vi "AAL Resample (Const to Variable, multi-channel).vi"(7 "reset? (True)":bool=TRUE, 8 "error in (no error)":errorcluster, 9 "config":T1={"timing jitter"=enum."Interpolation", "anti-aliasing?"=TRUE, "filter prototype"={"coefficients"=[], "factor"=1}} {"filter prototype"."coefficients" format="%.2f"}, 10 "time":dbl[](array[numeric]) format="%.2f", 11 "X":dbl[][](array[numeric])) -> (0 "error out":errorcluster, 1 "offset":i32, 2 "time stamps":dbl[](array[numeric]) format="%.2f", 3 "Y":dbl[][](array[numeric]) format="%.2f")   [LabVIEW 2010, in "NI_AALPro.lvlib"]
doc: "Perform an arbitrary resampling on the input signal."
uses:
  NI_AALPro.lvlib
  lvanlys.dll
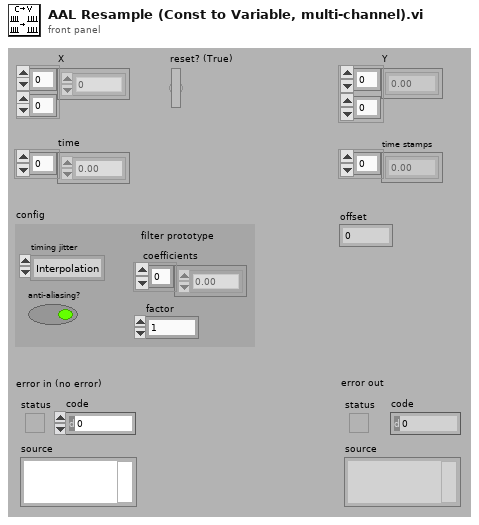
[diagram p1: front panel]
types:
  T1 = cluster{"timing jitter":enum32{"Interpolation", "Rounding"}, "anti-aliasing?":bool, "filter prototype":cluster{"coefficients":dbl[], "factor":i32}}
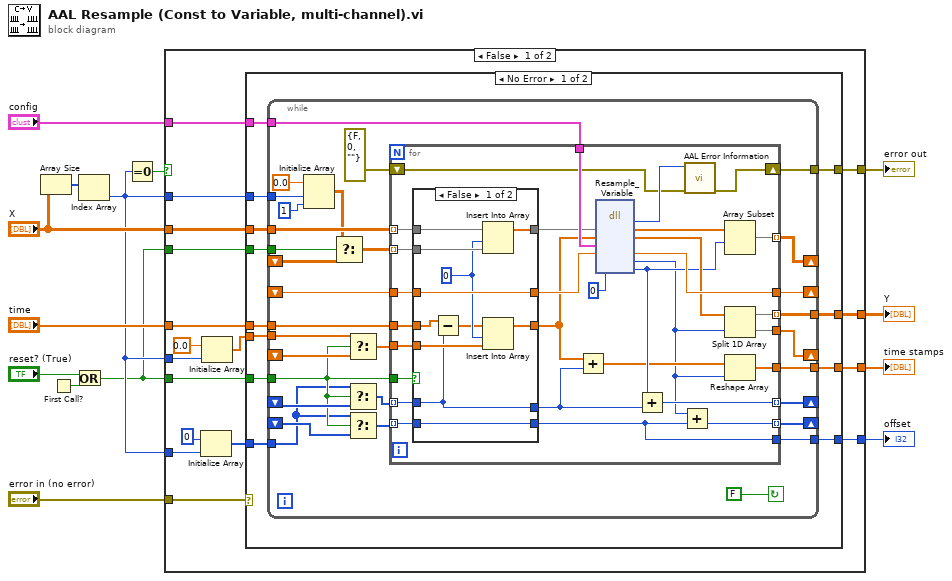
[diagram p0: block diagram]
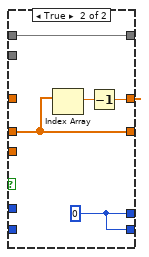
[diagram p2: hidden frame]
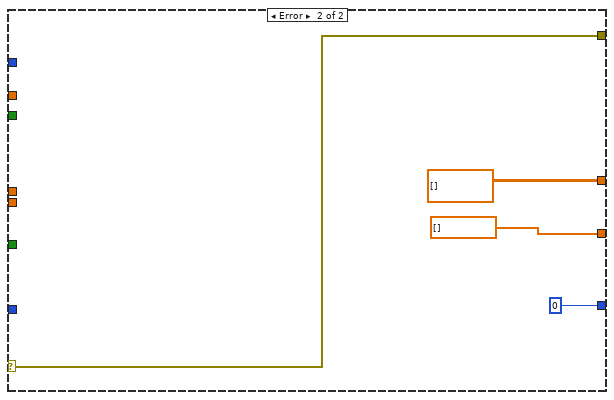
[diagram p3: hidden frame]
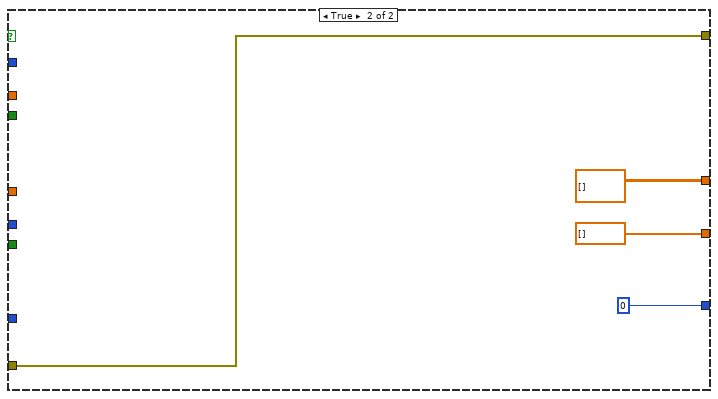
[diagram p4: hidden frame]
diagram:
  n1 = Array Size(array="X") -> (size(s)=w6:i32[])
  n2 = First Call?() -> (First Call?: T/F=w5:bool)
  n3 = Or(x="reset? (True)", y=w5) -> (x .or. y?=w1:bool)
  n4 = Index Array(array=w6) -> (element=w2:i32)  [unwired: 1 in]
  n5 = Equal To 0?(x=w2) -> (x = 0?=w3:bool)
  n6 = case shown="False" w3 {
    tunnel: "config" -> [w31 _]
    tunnel: "time" -> [w30 _]
    tunnel: [w29 dbl[] []] -> w12
    tunnel: [w28 dbl[][] []] -> w11
    tunnel: [w27 0 ("element")] -> w10
    tunnel: [w26 w126] -> w9
    tunnel: "error in (no error)" -> [w25 w126]
    tunnel: "X" -> [w24 _]
    tunnel: w1 -> [w21 _]
    tunnel: w2 -> [w19 _]
    tunnel: w2 -> [w17 _]
    tunnel: w2 -> [w16 _]
    tunnel: w1 -> [w15 _]
    frame False {
      n7 = Initialize Array(0 ("element"), w16) -> (w18:i32[])
      n8 = Initialize Array(0.0 ("element"), w17) -> (w20:dbl[])
      n9 = case shown="No Error" w25 {
        selector: w25 -> [_ w124]
        tunnel: w31 -> [w43 _]
        tunnel: w30 -> [w38 _]
        tunnel: [w42 dbl[] []] -> w29
        tunnel: [w41 dbl[][] []] -> w28
        tunnel: [w40 0] -> w27
        tunnel: [w39 w124] -> w26
        tunnel: w24 -> [w37 _]
        tunnel: w21 -> [w36 _]
        tunnel: w19 -> [w35 _]
        tunnel: w15 -> [w34 _]
        tunnel: w20 -> [w33 _]
        tunnel: w18 -> [w32 _]
        frame No Error {
          n10 = while {
            tunnel: [w66] -> w41
            tunnel: [w62] -> w42
            shift-right: [w72] -> _
            shift-left: _ -> [w52]
            shift-right: [w73] -> _
            shift-left: _ -> [w57]
            tunnel: w37 -> [w69]
            tunnel: w38 -> [w68]
            shift-right: [w71] -> _
            shift-left: _ -> [w67]
            tunnel: w36 -> [w45]
            tunnel: w43 -> [w74]
            shift-right: [w65] -> _
            shift-left: _ -> [w46]
            tunnel: [w64] -> w40
            shift-right: [w63] -> _
            shift-left: _ -> [w48]
            tunnel: [w60] -> w39
            tunnel: w34 -> [w58]
            tunnel: w35 -> [w53]
            tunnel: w33 -> [w50]
            tunnel: w32 -> [w44]
            stop <- FALSE continue-if-true
            n11 = Initialize Array(0.0, w53, 1 ("dimension size")) -> (w54:dbl[][])
            n12 = Select(t=w54, s=w58, f=w57) -> (s? t:f=w59:dbl[][])
            n13 = Select(t=w50, s=w45, f=w52) -> (s? t:f=w51:dbl[])
            n14 = Select(t=w44, s=w45, f=w46) -> (s? t:f=w47:i32[])
            n15 = Select(t=w44, s=w45, f=w48) -> (s? t:f=w49:i32[])
            n16 = for {
              tunnel: w74 -> [w104]
              tunnel: [w103] -> w73 mode=indexing
              tunnel: [w102] -> w72
              tunnel: [w101] -> w71
              tunnel: w69 -> [w100] mode=indexing
              tunnel: w68 -> [w98]
              tunnel: w59 -> [w96] mode=indexing
              tunnel: w51 -> [w95]
              tunnel: w67 -> [w94]
              tunnel: w45 -> [w93]
              tunnel: w47 -> [w91] mode=indexing
              tunnel: [w90] -> w66 mode=indexing
              tunnel: [w88] -> w65 mode=indexing
              tunnel: w49 -> [w83] mode=indexing
              tunnel: [w80] -> w64
              tunnel: [w79] -> w63 mode=indexing
              tunnel: [w77] -> w62
              shift-right: [w75] -> w60
              shift-left: errorcluster {"status"=FALSE, "code"=0, "source"=""} ("error out") -> [w76]
              w85 = 0
              n17 = case shown="False" w93 {
                tunnel: [w114 w120] -> w99
                tunnel: w100 -> [w112 w120]
                tunnel: [w109 w119] -> w87
                tunnel: w98 -> [w108 w119]
                tunnel: [w115 w117] -> w97
                tunnel: w96 -> [w111 _]
                tunnel: w95 -> [w113 _]
                tunnel: w94 -> [w115 _]
                tunnel: w91 -> [w106 _]
                tunnel: [w106 w116] -> w81
                tunnel: w83 -> [w105 _]
                tunnel: [w105 w116] -> w80
                frame False {
                  w110 = 0 ("Index")
                  n18 = Subtract(x=w108, y=w106) -> (x-y=w107:dbl[])
                  n19 = Insert Into Array(array=w112, index=w110, new element=w111) -> (w114:dbl[])
                  n20 = Insert Into Array(array=w107, index=w110, new element=w113) -> (w109:dbl[])
                }
                frame True {
                  w116 = 0
                  n21 = Index Array(array=w119) -> (element=w118:dbl)  [unwired: 1 in]
                  n22 = Decrement(x=w118) -> (x-1=w117:dbl)
                }
              }
              n23 = Add(x=w87, y=w81) -> (x+y=w86:dbl[])
              n24 = dll-call lib="C:/Program Files/National Instruments/LabVIEW 2010/resource/lvanlys.*" fn="Resample_Variable"("xH"=w99, "timeH"=w87, "config"=w104, "last_sample_time"=w97, "out_len"=w85, "xLeftOverIdx"=w85) -> (w78:i32, "xH"=w84:dbl[], "timeH"=w92:dbl[], "last_sample_time"=w101:dbl, "out_len"=w82:i32, "xLeftOverIdx"=w89:i32)  [unwired: 4 in, 2 out]
              n25 = Add(x=w89, y=w81) -> (x+y=w88:i32)
              n26 = Add(x=w82, y=w80) -> (x+y=w79:i32)
              n27 = call "AAL Error Information.vi"("error in (no error)"=w76, "error code"=w78) -> ("error out"=w75:errorcluster)  [unwired: 9 in]
              n28 = Array Subset(array=w84, index=w89) -> (w103:dbl[])  [unwired: 1 in]
              n29 = Split 1D Array(array=w92, index=w82) -> (first subarray=w90:dbl[], second subarray=w102:dbl[])
              n30 = Reshape Array(w86, w82) -> (w77:dbl[])
            }
          }
        }
        frame Error {
        }
      }
    }
    frame True {
    }
  }
  "time stamps" <- w12
  "Y" <- w11
  "offset" <- w10
  "error out" <- w9
